vi "Get_Symbol_Index.vi"(8 "error in (no error)":errorcluster, 11 "IB_TreeItem in":refnum<class "IB_Tree_Item.lvclass">) -> (0 "error out":errorcluster, 2 "symbol index":i32, 3 "IB_TreeItem out":refnum<class "IB_Tree_Item.lvclass">)   [LabVIEW 2020, in "IB_Tree_Item.lvclass"]
uses:
  <vilib>/AppBuilder/IB_Classes/Tree_Item/IB_Tree_Item.lvclass
  <vilib>/AppBuilder/IB_Classes/Tree_Item/IB_Tree_Item.lvclass/IB_Tree_Item.ctl
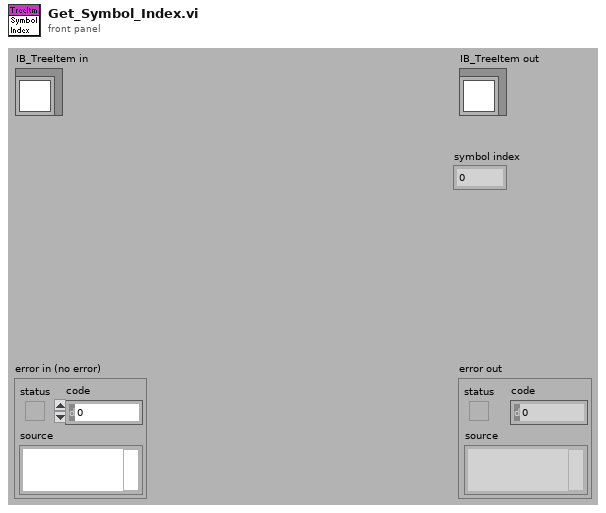
[diagram p1: front panel]
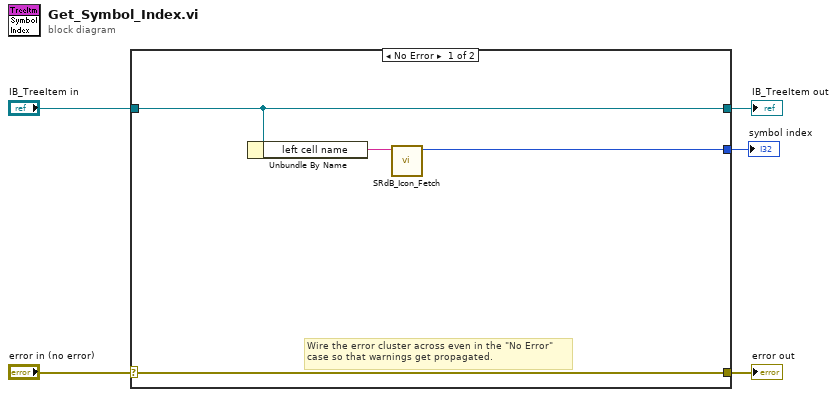
[diagram p0: block diagram]
diagram:
  n1 = case shown="No Error" "error in (no error)" {
    selector: "error in (no error)" -> [w9 w11]
    tunnel: [w9 w11] -> w4
    tunnel: [w8 w10] -> w2
    tunnel: "IB_TreeItem in" -> [w8 w10]
    tunnel: [w6 _] -> w1
    frame No Error {
      # "Wire the error cluster across even in the \"No Error\"\ncase so that warnings get propagated."
      n2 = Unbundle By Name(w8) -> ("left cell name"=w7:string)
      n3 = call <resource>:"SRdB_Icon_Fetch.vi"("filename"=w7) -> ("symbol index"=w6:i32)  [unwired: 8 in, 2 out]
    }
    frame Error {
    }
  }
  "error out" <- w4
  "IB_TreeItem out" <- w2
  "symbol index" <- w1
